vi "Generate_error.vi"(0 "Data_in":T2={"curr_h"=100.0, "curr_l"=0.0, "temp_h"=100.0, "temp_l"=0.0, "Acquiring?"=FALSE}, 5 "Current":dbl format="%#_13g", 7 "Temperature":dbl format="%#_13g", 11 "error in (no error)":errorcluster, 13 "Operations":T1=enum."Destroy") -> (4 "Error msg":refnum<user-event>, 15 "error IO":errorcluster)   [LabVIEW 2023, in "task_1.lvlib"]
doc: "Generate error by providing the current data and limits"
uses:
  task_1.lvlib
  Controls/data_limits.ctl
  Controls/event_operations.ctl
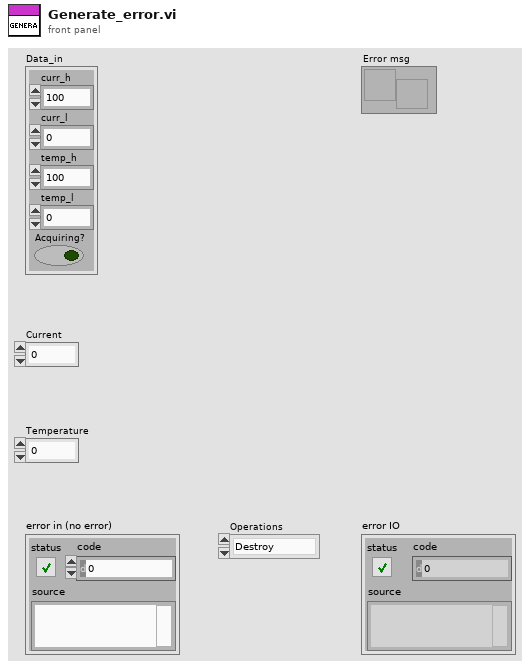
[diagram p1: front panel]
types:
  T1 = typedef "task_1.lvlib/event_operations.ctl" = enum16{"Create", "Generate", "Destroy"}
  T2 = typedef "task_1.lvlib/data_limits.ctl" = cluster{"curr_h":dbl, "curr_l":dbl, "temp_h":dbl, "temp_l":dbl, "Acquiring?":bool}
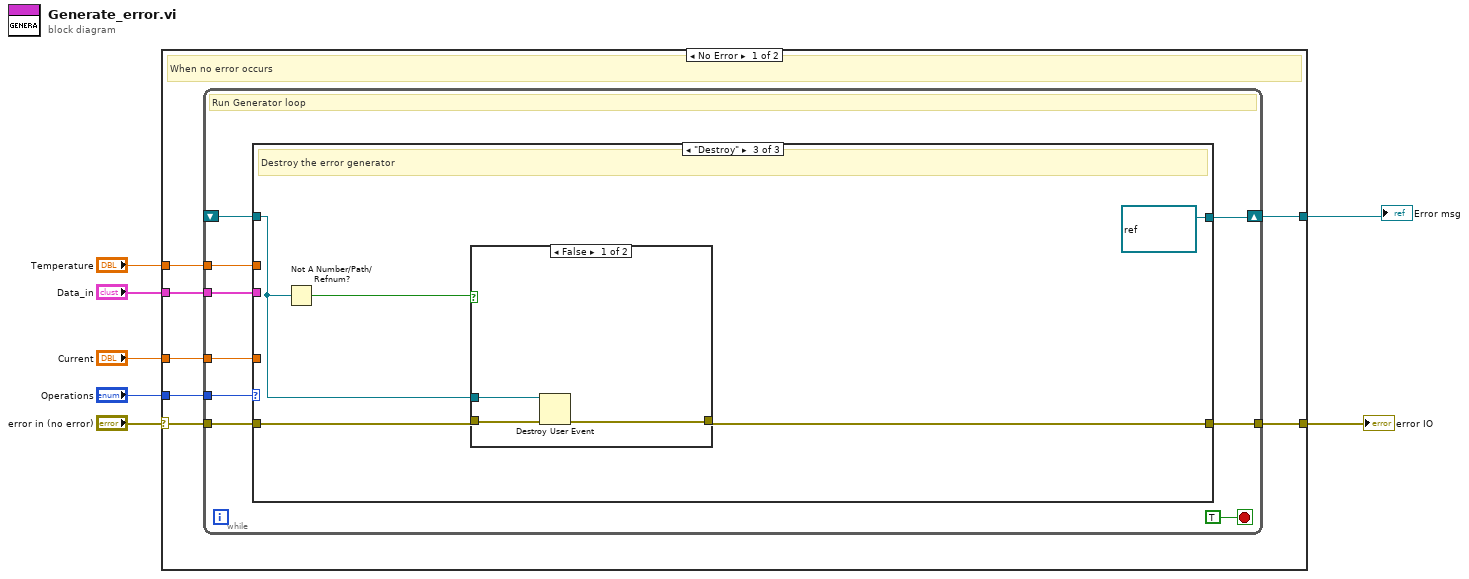
[diagram p0: block diagram]
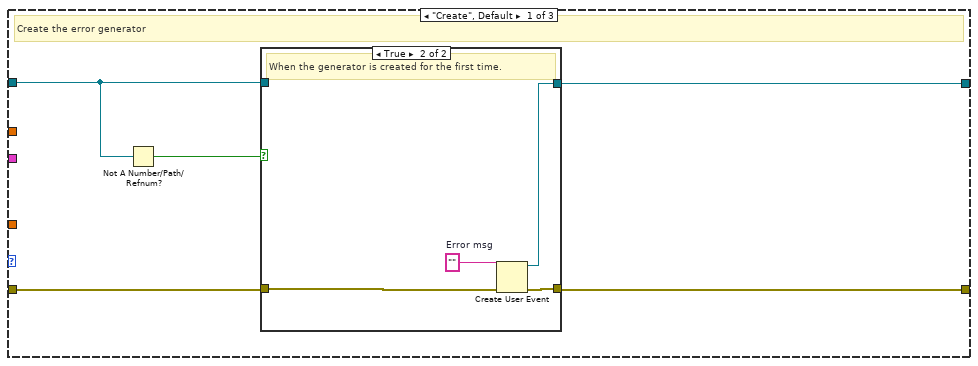
[diagram p2: hidden frame]
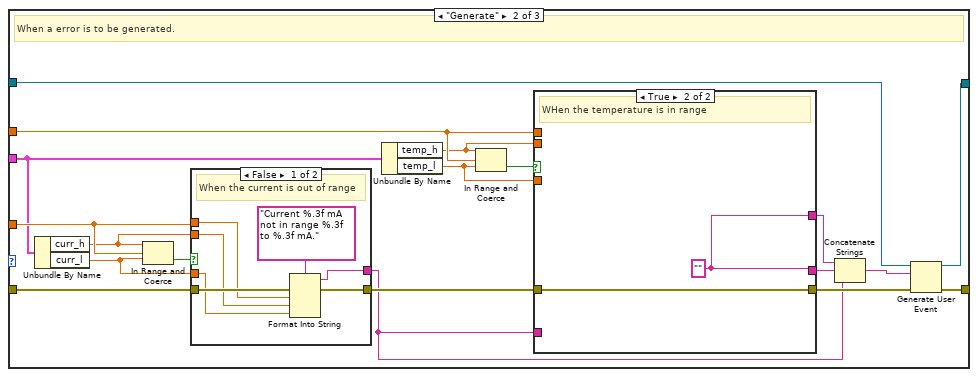
[diagram p4: hidden frame]
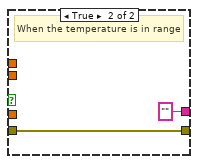
[diagram p5: hidden frame]
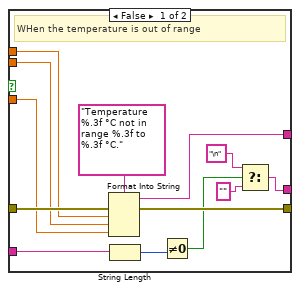
[diagram p6: hidden frame]
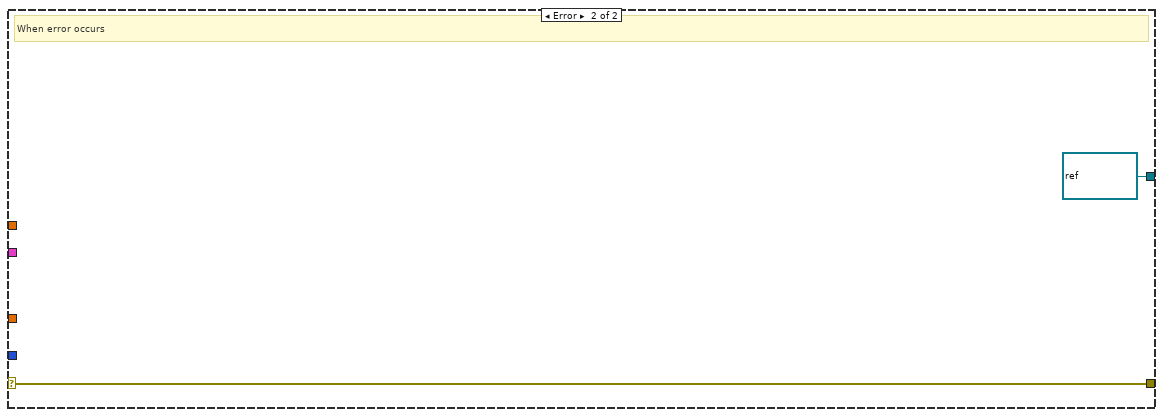
[diagram p8: hidden frame]
diagram:
  n1 = case shown="No Error" "error in (no error)" {
    selector: "error in (no error)" -> [w14 w88]
    tunnel: [w13 w88] -> w2
    tunnel: "Operations" -> [w12 _]
    tunnel: "Data_in" -> [w11 _]
    tunnel: "Current" -> [w10 _]
    tunnel: "Temperature" -> [w9 _]
    tunnel: [w8 refnum<user-event> refnum ("Error msg")] -> w1
    frame No Error {
      # "When no error occurs"
      n2 = while {
        tunnel: w14 -> [w23]
        tunnel: [w22] -> w13
        shift-right: [w20] -> w8
        shift-left: _ -> [w19]
        tunnel: w12 -> [w18]
        tunnel: w11 -> [w17]
        tunnel: w10 -> [w16]
        tunnel: w9 -> [w15]
        stop <- TRUE stop-if-true
        # "Run Generator loop"
        n3 = case shown="\"Destroy\"" w18 {
          tunnel: w23 -> [w28 w51 w81]
          tunnel: [w27 w41 w80] -> w22
          tunnel: [w26 w37 refnum<user-event> refnum ("Error msg")] -> w20
          tunnel: w19 -> [w24 w40 w79]
          tunnel: w17 -> [_ w46 _]
          tunnel: w16 -> [_ w52 _]
          tunnel: w15 -> [_ w44 _]
          frame "Create", Default {
            # "Create the error generator"
            n4 = Not A Number/Path/Refnum?(number/path/refnum=w24) -> (NaN/Path/Refnum?=w25:bool)
            n5 = case shown="True" w25 {
              tunnel: w28 -> [w30 w34]
              tunnel: [w30 w33] -> w27
              tunnel: [w29 w32] -> w26
              tunnel: w24 -> [w29 _]
              frame False {
                # "When the generator already exists"
              }
              frame True {
                w31 = ""  # Error msg
                # "When the generator is created for the first time."
                n6 = Create User Event(user event datatype=w31, error in=w34) -> (user event=w32:refnum<user-event>, error out=w33:errorcluster)
              }
            }
          }
          frame "Generate" {
            # "When a error is to be generated."
            n7 = Unbundle By Name(w46) -> ("curr_h"=w48:dbl, "curr_l"=w47:dbl)
            n8 = In Range and Coerce(upper limit=w48, x=w52, lower limit=w47) -> (In Range?=w53:bool)  [unwired: 1 out]
            n9 = case shown="False" w53 {
              tunnel: w52 -> [w57 _]
              tunnel: w51 -> [w60 w62]
              tunnel: [w59 w62] -> w50
              tunnel: w48 -> [w55 _]
              tunnel: w47 -> [w56 _]
              tunnel: [w54 ""] -> w35
              frame False {
                # "When the current is out of range"
                n10 = Format Into String(format string="Current %.3f mA not in range %.3f to %.3f mA.", error in=w60, w57, w55, w56) -> (resulting string=w54:string, error out=w59:errorcluster)  [unwired: 1 in]
              }
              frame True {
                # "When the temperature is in range"
              }
            }
            n11 = Unbundle By Name(w46) -> ("temp_h"=w43:dbl, "temp_l"=w42:dbl)
            n12 = In Range and Coerce(upper limit=w43, x=w44, lower limit=w42) -> (In Range?=w45:bool)  [unwired: 1 out]
            n13 = case shown="True" w45 {
              tunnel: w50 -> [w75 w77]
              tunnel: [w74 w77] -> w49
              tunnel: w44 -> [w72 _]
              tunnel: w43 -> [w71 _]
              tunnel: w42 -> [w70 _]
              tunnel: [w69 w76] -> w39
              tunnel: w35 -> [w68 _]
              tunnel: [w63 w76] -> w36
              frame False {
                # "WHen the temperature is out of range"
                n14 = Format Into String(format string="Temperature %.3f °C not in range %.3f to %.3f °C.", error in=w75, w72, w71, w70) -> (resulting string=w69:string, error out=w74:errorcluster)  [unwired: 1 in]
                n15 = String Length(string=w68) -> (length=w67:i32)
                n16 = Not Equal To 0?(x=w67) -> (x != 0?=w66:bool)
                n17 = Select(t="\n", s=w66, f="") -> (s? t:f=w63:string)
              }
              frame True {
                w76 = ""
                # "WHen the temperature is in range"
              }
            }
            n18 = Concatenate Strings(w39, w36, w35) -> (w38:string)
            n19 = Generate User Event(user event=w40, event data cluster=w38, error in=w49) -> (user event out=w37:refnum<user-event>, error out=w41:errorcluster)  [unwired: 1 in]
          }
          frame "Destroy" {
            # "Destroy the error generator"
            n20 = Not A Number/Path/Refnum?(number/path/refnum=w79) -> (NaN/Path/Refnum?=w82:bool)
            n21 = case shown="False" w82 {
              tunnel: w81 -> [w85 w86]
              tunnel: [w84 w86] -> w80
              tunnel: w79 -> [w83 _]
              frame False {
                n22 = Destroy User Event(user event=w83, error in=w85) -> (error out=w84:errorcluster)
              }
              frame True {
              }
            }
          }
        }
      }
    }
    frame Error {
      # "When error occurs"
    }
  }
  "error IO" <- w2
  "Error msg" <- w1
